vi "Write Buttons.vi"(10 "Buttons":T1, 11 "User Interface in":refnum<class "User Interface.lvclass">) -> (3 "User Interface out":refnum<class "User Interface.lvclass">)   [LabVIEW 2016, in "User Interface.lvlib" / "User Interface.lvclass"]
uses:
  User Interface.lvclass
  Buttons.ctl
  User Interface.lvlib
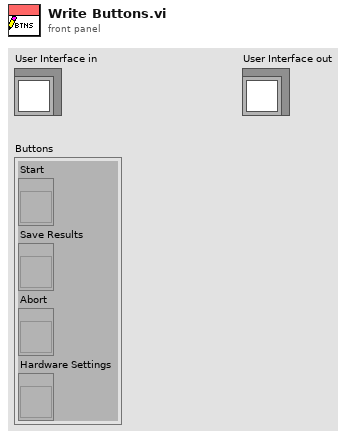
[diagram p1: front panel]
types:
  T1 = typedef "User Interface.lvlib/Buttons.ctl" = cluster{"Start":refnum<vi>, "Save Results":refnum<vi>, "Abort":refnum<vi>, "Hardware Settings":refnum<vi>}
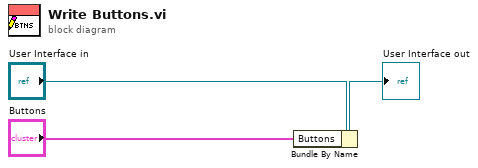
[diagram p0: block diagram]
diagram:
  n1 = Bundle By Name(cluster="User Interface in", "Buttons"="Buttons") -> (→"User Interface out":refnum<class "User Interface.lvclass">)
